vi "Exercise 3-7.vi"() -> ()   [LabVIEW 2014]
panel:
  out "Sqaure Root value":dbl
  in  "Numeric":dbl
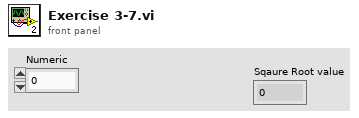
[diagram p1: front panel]
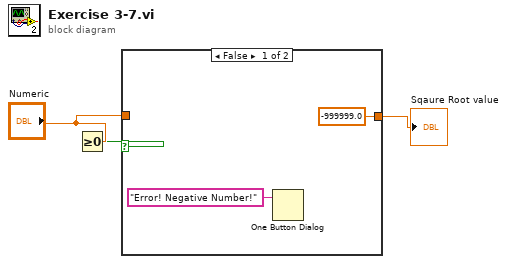
[diagram p0: block diagram]
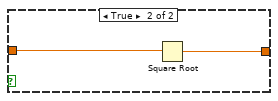
[diagram p2: hidden frame]
diagram:
  n1 = Greater Or Equal To 0?(x="Numeric") -> (x >= 0?=w1:bool)
  n2 = case shown="False" w1 {
    tunnel: "Numeric" -> [_ w7]
    tunnel: [-999999.0 w6] -> w2
    frame False {
      n3 = One Button Dialog(message="Error! Negative Number!") -> ()  [unwired: 1 in, 1 out]
    }
    frame True {
      n4 = Square Root(x=w7) -> (sqrt(x)=w6:dbl)
    }
  }
  "Sqaure Root value" <- w2
